vi "Average_angles_student.vi"(10 "Angle_2":dbl, 11 "Angle_1":dbl) -> (3 "Angle_average":dbl)   [LabVIEW 2014]
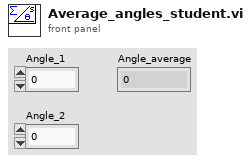
[diagram p1: front panel]
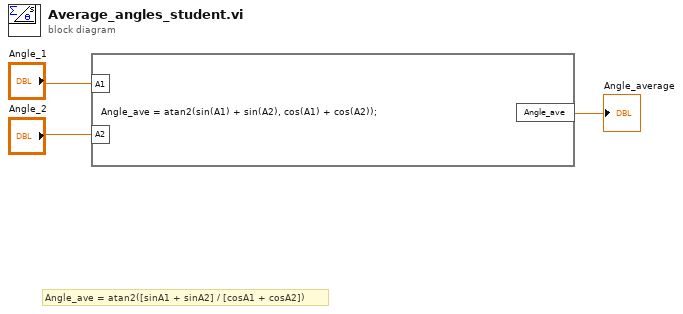
[diagram p0: block diagram]
diagram:
  # "Angle_ave = atan2([sinA1 + sinA2] / [cosA1 + cosA2])"
  n1 = formula code="Angle_ave = atan2(sin(A1) + sin(A2), cos(A1) + cos(A2));"("A1"="Angle_1", "A2"="Angle_2") -> ("Angle_ave"=→"Angle_average":dbl)
